vi "Sequence Check Next RPM.vi"(11 "Sequencer Data Context IN":T1={"Sequencer State"=enum."Idle", "Event Timeout"=-1, "Current Index"=0, "Sequence Timeout"=0, "Turbine RPM Array"=[], "Pump RPM Array"=[], "Duration (Seconds) Array"=[]}) -> (3 "Sequencer Data Context OUT":T1={"Sequencer State"=enum."Idle", "Event Timeout"=-1, "Current Index"=0, "Sequence Timeout"=0, "Turbine RPM Array"=[], "Pump RPM Array"=[], "Duration (Seconds) Array"=[]})   [LabVIEW 2024, in "Auto Modo.lvlib"]
uses:
  Auto Modo.lvlib
  Sequencer State.ctl
  Sequencer Data Context.ctl
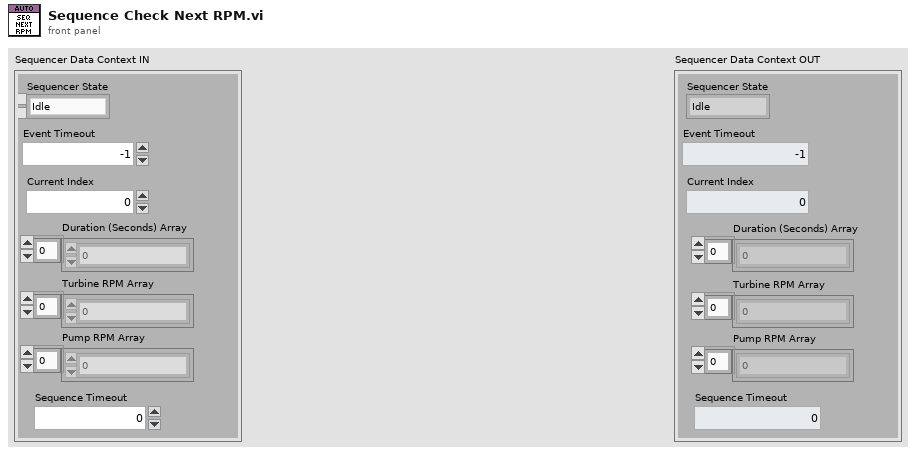
[diagram p1: front panel]
types:
  T1 = typedef "Auto Modo.lvlib/Sequencer Data Context.ctl" = cluster{"Sequencer State":T2, "Event Timeout":i32, "Current Index":i32, "Sequence Timeout":i32, "Turbine RPM Array":dbl[], "Pump RPM Array":dbl[], "Duration (Seconds) Array":dbl[]}
  T2 = typedef "Auto Modo.lvlib/Sequencer State.ctl" = enum16{"Idle", "Clear Drive Fault", "Check Drive Fault", "Set Ready to Switch ON", "Check Ready to Switch ON", "Enable Operation", "Check Enable Operation", "Set Drive RPM", "Check Drive RPM", "Next Drive RPM", "Final"}
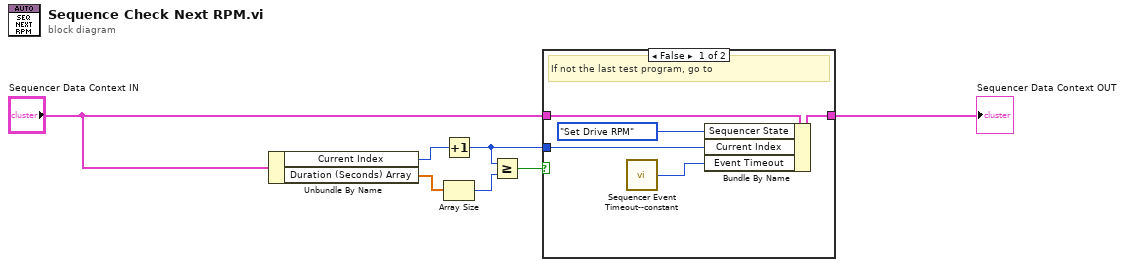
[diagram p0: block diagram]
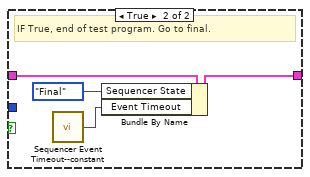
[diagram p2: hidden frame]
diagram:
  n1 = Unbundle By Name("Sequencer Data Context IN") -> ("Current Index"=w6:i32, "Duration (Seconds) Array"=w7:dbl[])
  n2 = Increment(x=w6) -> (x+1=w1:i32)
  n3 = Array Size(array=w7) -> (size(s)=w5:i32)
  n4 = Greater Or Equal?(x=w1, y=w5) -> (x >= y?=w4:bool)
  n5 = case shown="False" w4 {
    tunnel: "Sequencer Data Context IN" -> [w11 w16]
    tunnel: [w10 w15] -> w3
    tunnel: w1 -> [w8 _]
    frame False {
      # "If not the last test program, go to"
      n6 = call "Sequencer Event Timeout--constant.vi"() -> ("Event Timeout (ms)"=w9:i32)  [unwired: 1 in]
      n7 = Bundle By Name(cluster=w11, "Sequencer State"=Sequencer_State."Set Drive RPM", "Current Index"=w8, "Event Timeout"=w9) -> (w10:T1)
    }
    frame True {
      # "IF True, end of test program. Go to final."
      n8 = call "Sequencer Event Timeout--constant.vi"() -> ("Event Timeout (ms)"=w14:i32)  [unwired: 1 in]
      n9 = Bundle By Name(cluster=w16, "Sequencer State"=Sequencer_State."Final", "Event Timeout"=w14) -> (w15:T1)
    }
  }
  "Sequencer Data Context OUT" <- w3
